vi "CRYGet Tree Reference.vi"(10 "Label Name":string, 11 "VI Refnum":refnum<vi>) -> (1 "Find?":bool, 2 "Tree Ref Out":refnum<vi>, 3 "VI Refnum Out":refnum<vi>)   [LabVIEW 2013]
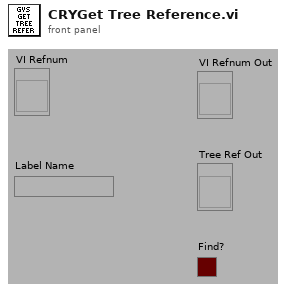
[diagram p1: front panel]
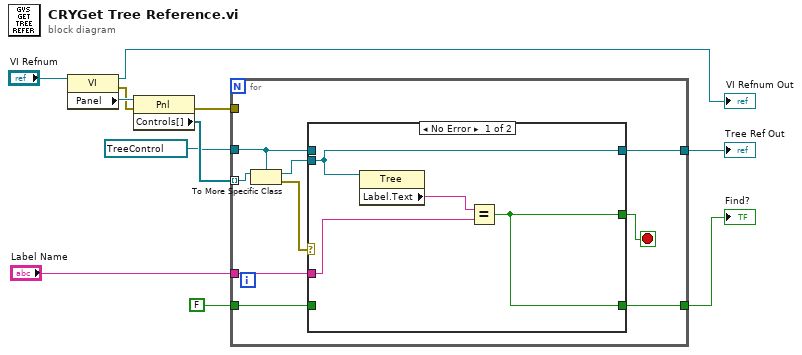
[diagram p0: block diagram]
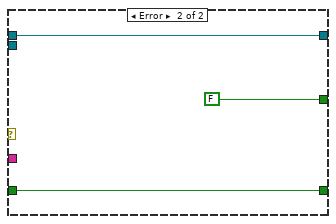
[diagram p2: hidden frame]
diagram:
  n1 = property class="VI"(reference="VI Refnum") -> (reference out=→"VI Refnum Out":refnum<vi>, error out=w2:errorcluster, "Panel"=w4:refnum<vi>)  [unwired: 1 in]
  n2 = property class="Pnl"(reference=w4, error in=w2) -> (error out=w1:errorcluster, "Controls[]"=w10:refnum<vi>[])  [unwired: 1 out]
  n3 = for {
    tunnel: w10 -> [w20] mode=indexing
    tunnel: [w16] -> w7
    tunnel: "Label Name" -> [w15]
    tunnel: refnum<vi> refnum ("ControlType") -> [w14]
    tunnel: FALSE ("Boolean") -> [w13]
    tunnel: [w12] -> w5
    tunnel: w1 -> [_]
    stop <- w17 stop-if-true
    n4 = To More Specific Class(target class=w14, reference=w20) -> (specific class reference=w18:refnum<vi>, error out=w19:errorcluster)  [unwired: 1 in]
    n5 = case shown="No Error" w19 {
      tunnel: w18 -> [w22 _]
      tunnel: [w21 FALSE] -> w17
      tunnel: [w22 w26] -> w16
      tunnel: w15 -> [w23 _]
      tunnel: w14 -> [_ w26]
      tunnel: [w21 w25] -> w12
      tunnel: w13 -> [_ w25]
      frame No Error {
        n6 = property class="Tree"(reference=w22) -> ("Label.Text"=w24:string)  [unwired: 1 in, 2 out]
        n7 = Equal?(x=w24, y=w23) -> (x = y?=w21:bool)
      }
      frame Error {
      }
    }
  }
  "Find?" <- w5
  "Tree Ref Out" <- w7
